vi "Create Evaluation String.vi"(8 "error in (no error)":errorcluster, 10 "Evaluation String":string, 11 "Int Equal in":refnum<class "Int Equal.lvclass">) -> (0 "error out":errorcluster, 3 "Int Equal out":refnum<class "Int Equal.lvclass">)   [LabVIEW 2018, in "Int Equal.lvclass"]
uses:
  Int Equal.lvclass
  C:/Users/UKHornP/Documents/Work/Projects/Assert API/Plugins/Utility/Test Classes/Test.lvclass
  Integer.lvclass
  Test.lvclass
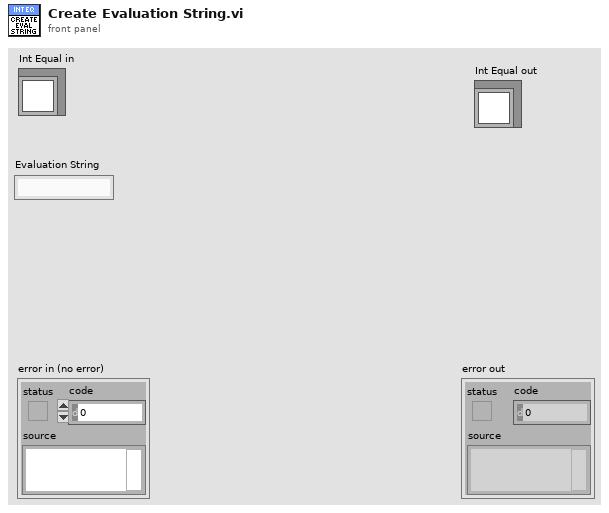
[diagram p1: front panel]
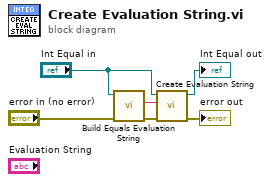
[diagram p0: block diagram]
diagram:
  n1 = call "Build Equals Evaluation String.vi"("error in (no error)"="error in (no error)", "Test in"="Int Equal in") -> ("error out"=w3:errorcluster, "Equals Evaluation String"=w1:string)  [unwired: 8 in]
  n2 = call-parent "Create Evaluation String.vi"("error in (no error)"=w3, "Evaluation String"=w1, "Integer in"="Int Equal in") -> ("error out"=→"error out":errorcluster, "Integer out"=→"Int Equal out":refnum<class "Int Equal.lvclass">)  [unwired: 7 in]
